vi "FV-View-miniVNA_multifile.vi"() -> ()   [LabVIEW 2020, in "FV-file_viewer.lvlib"]
uses:
  FV-file_viewer.lvlib
  record_file_handler/VFH-VNA_File_Handler.lvlib
panel:
  out "Array 4":errorcluster[](array[cluster])
  out "Array 3":bool[](array[boolean])
  out "Array 2":path[](array[path])
  out "Magnitude":cluster{"Frequency":dbl[], "S21_Imag":dbl[]}[](graph)
  out "S11 R":cluster{"Frequency":dbl[], "S21_Imag":dbl[]}[](graph)
  out "|Z|":cluster{"Frequency":dbl[], "S21_Imag":dbl[]}[](graph)
  out "S11 I":cluster{"Frequency":dbl[], "S21_Imag":dbl[]}[](graph)
  out "Cluster":T1 {"Z''" format="%#_5p"; "Z'" format="%#_5p"; "|Z|" format="%#_5p"; "Loss" format="%#_5p"; "Deg" format="%#_5p"; "Phi" format="%#_5p"; "Mag" format="%#_5p"; "S11 I" format="%#_5p"; "S11 R" format="%#_5p"}
  in  "index":i32
  out "Freq":dbl format="%#_6p"
  out "Array":dbl[](array[numeric]) format="%#_5p"
  in  "Signal":i32
  in  "Stop":bool
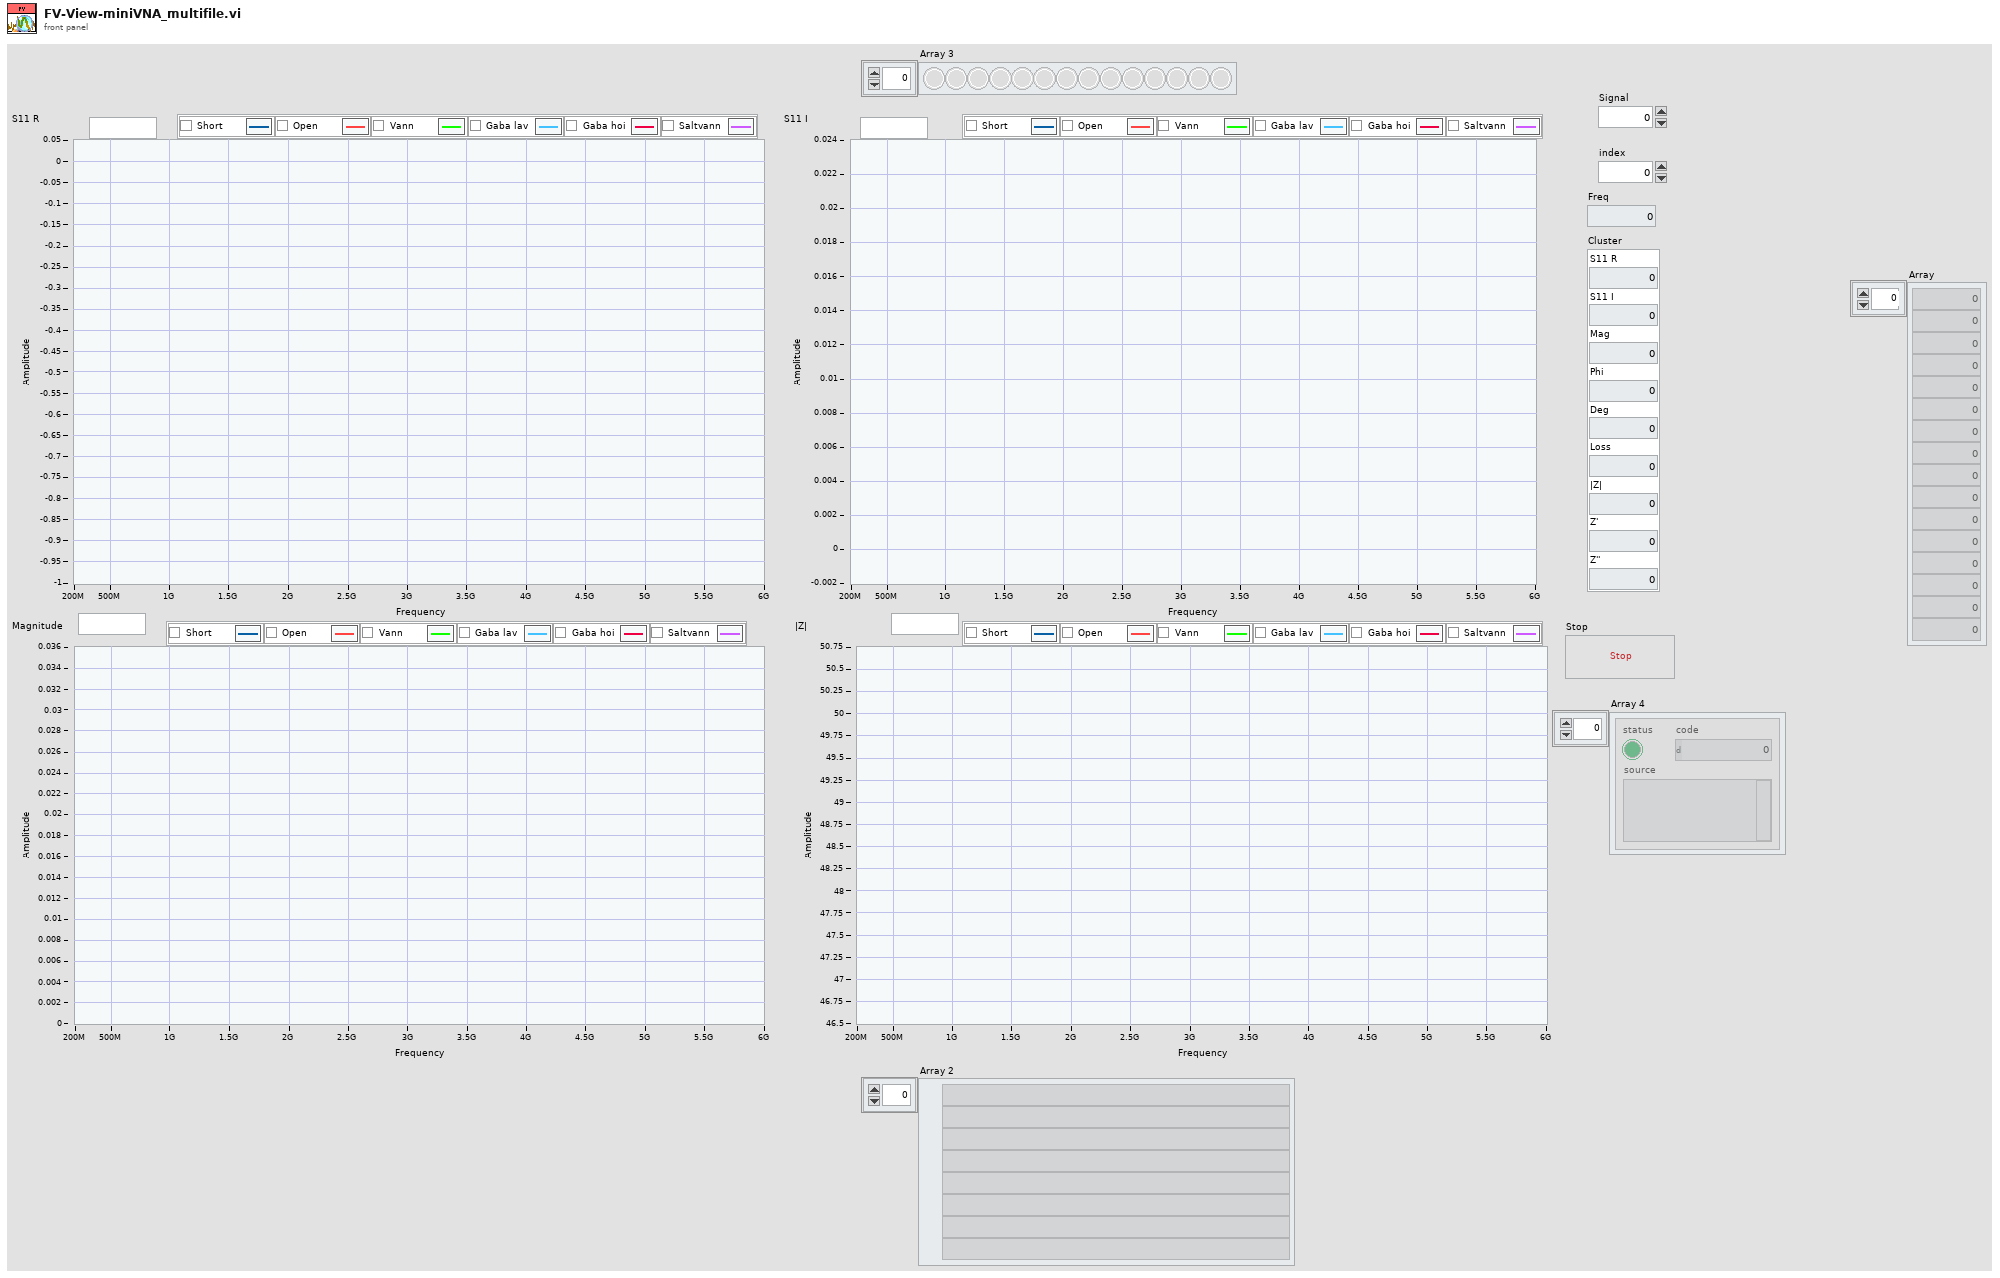
[diagram p1: front panel]
types:
  T1 = cluster{"S11 R":dbl, "S11 I":dbl, "Mag":dbl, "Phi":dbl, "Deg":dbl, "Loss":dbl, "|Z|":dbl, "Z'":dbl, "Z''":dbl}
  T2 = typedef "VFH-VNA_File_Handler.lvlib/VFH-file_cluster-NanoVNA.ctl" = cluster{"Frequency":dbl[], "S11_Real":dbl[], "S11_Imag":dbl[], "S21_Real":dbl[], "S21_Imag":dbl[], "S12_Real":dbl[], "S12_Imag":dbl[], "S22_Real":dbl[], "S22_Imag":dbl[]}
  T3 = cluster{"Loss":cluster{"Frequency":dbl[], "Array":dbl[]}, "Z Modulus":cluster{"Frequency":dbl[], "Array":dbl[]}, "Z'":cluster{"Frequency":dbl[], "Array":dbl[]}, "Z''":cluster{"Frequency":dbl[], "Array":dbl[]}}
  T4 = cluster{"S11'":cluster{"Frequency":dbl[], "S11_Real":dbl[]}, "S11''":cluster{"Frequency":dbl[], "S11_Real":dbl[]}, "Magnitude":cluster{"Frequency":dbl[], "Array":dbl[]}, "Eta":cluster{"Frequency":dbl[], "Array":dbl[]}, "Phase":cluster{"Frequency":dbl[], "Array":dbl[]}}
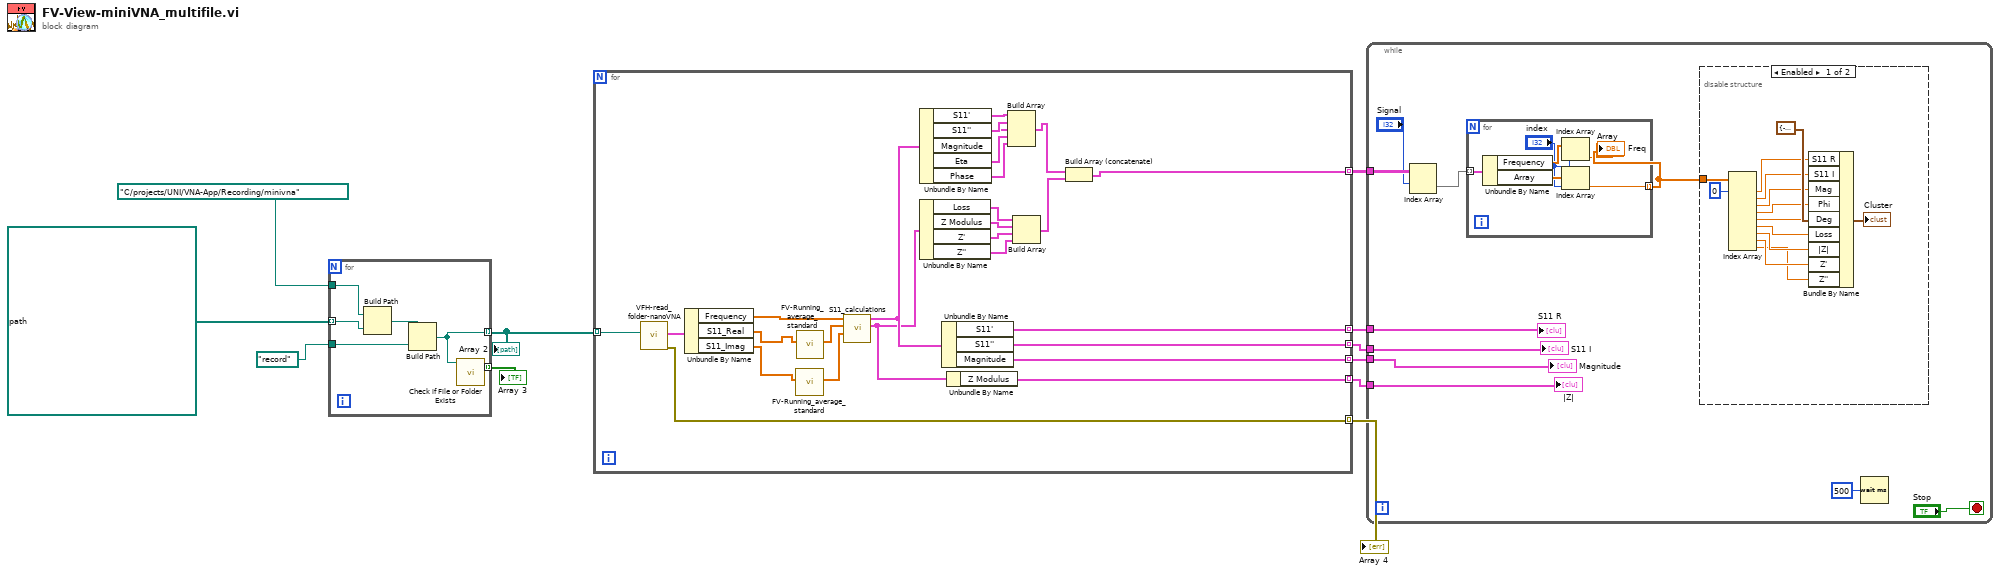
[diagram p0: block diagram]
diagram:
  n1 = for {
    tunnel: path[] [path "test-short", path "test-open", path "test-Vann", path "test-Gabalav", path "test-gabahøy", path "test-Saltvann"] ("Folder Path") -> [w16] mode=indexing
    tunnel: path "C:/projects/UNI/VNA-App/Recording/minivna" ("Folder Path") -> [w17]
    tunnel: [w13] -> w4 mode=indexing
    tunnel: [w15] -> w3 mode=indexing
    tunnel: path "record" ("name or relative path") -> [w12]
    n2 = Build Path(base path=w17, name or relative path=w16) -> (appended path=w14:path)
    n3 = Build Path(base path=w14, name or relative path=w12) -> (appended path=w13:path)
    n4 = call <vilib>:"Check if File or Folder Exists.vi"("path"=w13) -> ("file or folder exists?"=w15:bool)  [unwired: 8 in, 2 out]
  }
  "Array 2" <- w4
  "Array 3" <- w3
  n5 = for {
    tunnel: w4 -> [w29] mode=indexing
    tunnel: [w27] -> w11 mode=indexing
    tunnel: [w26] -> w10 mode=indexing
    tunnel: [w25] -> w8 mode=indexing
    tunnel: [w24] -> w9 mode=indexing
    tunnel: [w23] -> w7 mode=indexing
    tunnel: [w22] -> w1 mode=indexing
    n6 = call "VFH-read_folder-nanoVNA.vi"("Folder Path"=w29) -> ("error out"=w22:errorcluster, "avg output"=w28:T2)  [unwired: 7 in, 2 out]
    n7 = Unbundle By Name(w28) -> ("Frequency"=w43:dbl[], "S11_Real"=w21:dbl[], "S11_Imag"=w19:dbl[])
    n8 = call "FV-Running_average_standard.vi"("in"=w19) -> ("Out"=w18:dbl[])  [unwired: 10 in]
    n9 = call "FV-Running_average_standard.vi"("in"=w21) -> ("Out"=w20:dbl[])  [unwired: 10 in]
    n10 = call "S11_calculations.vi"("S11_Imag"=w18, "S11_Real"=w20, "Frequency"=w43) -> ("Calc"=w30:T3, "Raw"=w31:T4)  [unwired: 6 in, 1 out]
    n11 = Unbundle By Name(w31) -> ("S11'"=w42:cluster{"Frequency":dbl[], "S11_Real":dbl[]}, "S11''"=w41:cluster{"Frequency":dbl[], "S11_Real":dbl[]}, "Magnitude"=w40:cluster{"Frequency":dbl[], "Array":dbl[]}, "Eta"=w39:cluster{"Frequency":dbl[], "Array":dbl[]}, "Phase"=w38:cluster{"Frequency":dbl[], "Array":dbl[]})
    n12 = Unbundle By Name(w30) -> ("Loss"=w37:cluster{"Frequency":dbl[], "Array":dbl[]}, "Z Modulus"=w36:cluster{"Frequency":dbl[], "Array":dbl[]}, "Z'"=w35:cluster{"Frequency":dbl[], "Array":dbl[]}, "Z''"=w34:cluster{"Frequency":dbl[], "Array":dbl[]})
    n13 = Unbundle By Name(w31) -> ("S11'"=w27:cluster{"Frequency":dbl[], "S11_Real":dbl[]}, "S11''"=w26:cluster{"Frequency":dbl[], "S11_Real":dbl[]}, "Magnitude"=w25:cluster{"Frequency":dbl[], "Array":dbl[]})
    n14 = Unbundle By Name(w30) -> ("Z Modulus"=w24:cluster{"Frequency":dbl[], "Array":dbl[]})
    n15 = Build Array(w42, w41, w40, w39, w38) -> (w32:cluster{"Frequency":dbl[], "Array":dbl[]}[])
    n16 = Build Array(w37, w36, w35, w34) -> (w33:cluster{"Frequency":dbl[], "Array":dbl[]}[])
    n17 = Build Array (concatenate)(w32, w33) -> (w23:cluster{"Frequency":dbl[], "Array":dbl[]}[])
  }
  "Array 4" <- w1
  n18 = while {
    tunnel: w11 -> [w53]
    tunnel: w10 -> [w52]
    tunnel: w9 -> [w51]
    tunnel: w8 -> [w50]
    tunnel: w7 -> [w48]
    stop <- "Stop" stop-if-true
    n19 = Index Array(array=w48, index (row)="Signal") -> (element=w47:cluster{"Frequency":dbl[], "Array":dbl[]}[])  [unwired: 1 in]
    n20 = for {
      tunnel: w47 -> [w59] mode=indexing
      tunnel: [w54] -> w49 mode=indexing
      n21 = Unbundle By Name(w59) -> ("Frequency"=w57:dbl[], "Array"=w58:dbl[])
      n22 = Index Array(array=w57, index="index") -> (element=→"Freq":dbl)
      n23 = Index Array(array=w58, index="index") -> (element=w54:dbl)
    }
    "Array" <- w49
    n24 = disable-structure shown="Enabled" {
      disable-tunnel: w49 -> [w72 _]
      frame Enabled {
        n25 = Index Array(array=w72, index #1=0 ("index (row)")) -> (element #1=w69:dbl, element #2=w68:dbl, element #3=w67:dbl, element #4=w66:dbl, element #5=w65:dbl, element #6=w64:dbl, element #7=w63:dbl, element #8=w62:dbl, element #9=w61:dbl)  [unwired: 8 in]
        n26 = Bundle By Name(cluster=T1 {"S11 R"=-0.13079270605384616, "S11 I"=-0.13079270605384616, "Mag"=-0.13079270605384616, "Phi"=-0.13079270605384616, "Deg"=-0.13079270605384616, "Loss"=-0.13079270605384616, "|Z|"=-0.13079270605384616, "Z'"=-0.13079270605384616, "Z''"=-0.13079270605384616} ("Cluster"), "S11 R"=w69, "S11 I"=w68, "Mag"=w67, "Phi"=w66, "Deg"=w65, "Loss"=w64, "|Z|"=w63, "Z'"=w62, "Z''"=w61) -> (→"Cluster":T1)
      }
      frame Disabled {
      }
    }
    n27 = Wait (ms)(milliseconds to wait=u32 500) -> ()  [unwired: 1 out]
    "Magnitude" <- w50
    "S11 R" <- w53
    "|Z|" <- w51
    "S11 I" <- w52
  }
